vi "neuronFound.vi"(6 "Pipette broken threshold (MOhms)":dbl=-0.5, 8 "NH method":T1, 9 "Extra threshold (MOhms)":dbl=0.15, 10 "Detection Threshold (MOhms)":dbl=0.05, 11 "R array":dbl[](array[numeric])) -> (2 "pipette broken - abort!":bool, 3 "neuron found":bool)   [LabVIEW 2015]
uses:
  <vilib>/Analysis/NI_AALBase.lvlib
  <vilib>/Analysis/baseanly.llb/Mean (DBL).vi
  controls/NH_method.ctl
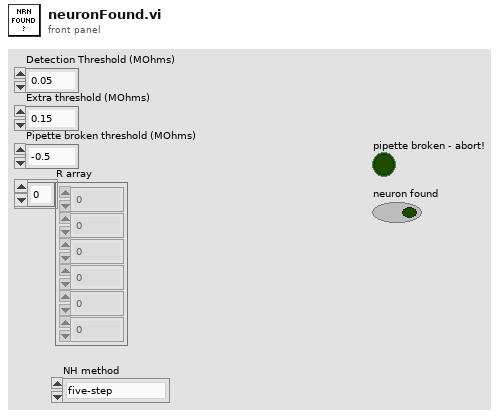
[diagram p1: front panel]
types:
  T1 = typedef "NH_method.ctl" = enum16{"five-step", "three-stepANDfixedCutOff", "three-step"}
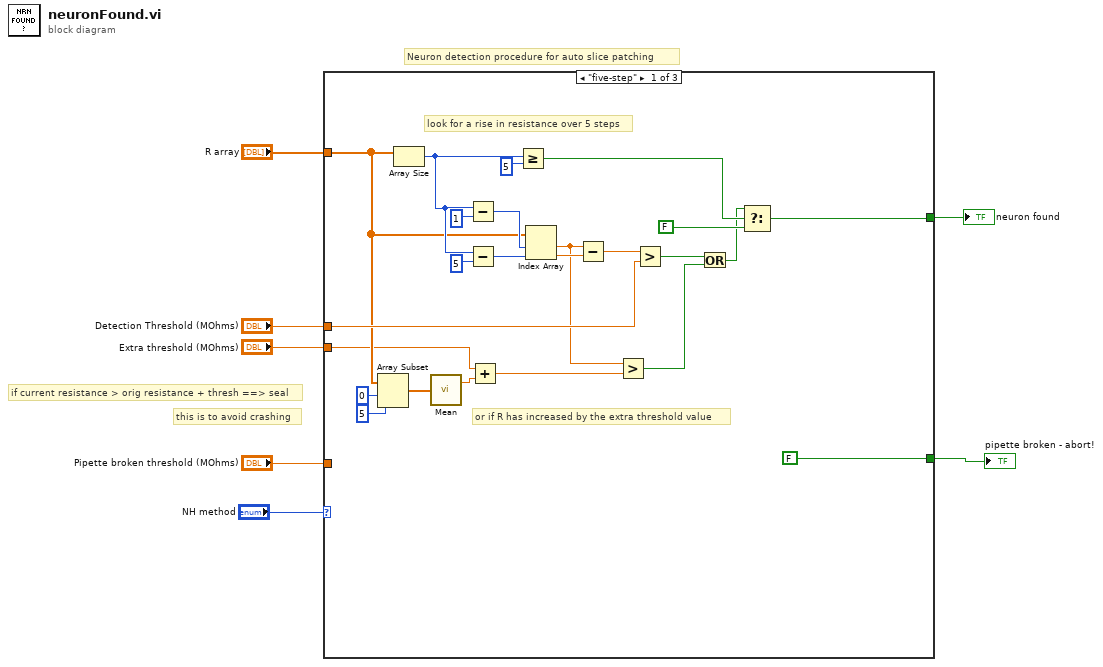
[diagram p0: block diagram]
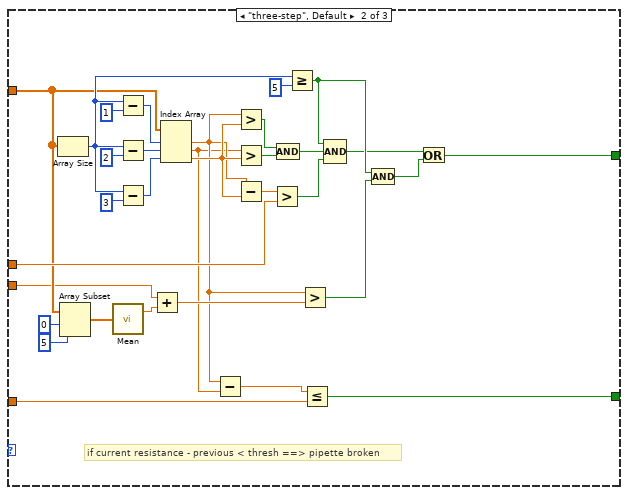
[diagram p2: hidden frame]
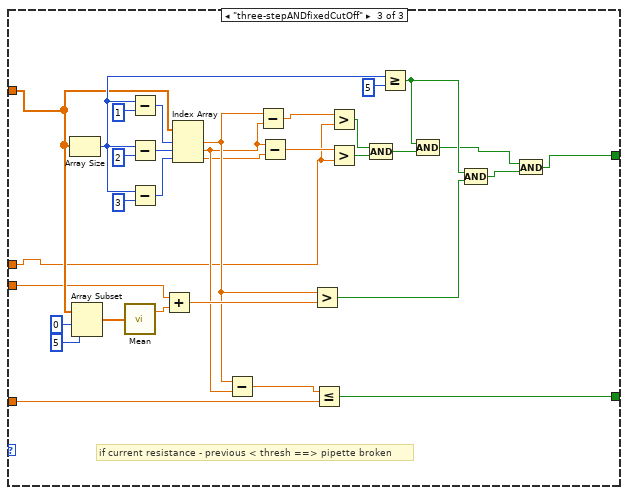
[diagram p3: hidden frame]
diagram:
  # "this is to avoid crashing"
  # "if current resistance > orig resistance + thresh ==> seal"
  # "Neuron detection procedure for auto slice patching"
  n1 = case shown="\"five-step\"" "NH method" {
    tunnel: [w20 w39 w64] -> w7
    tunnel: "R array" -> [w13 w48 w75]
    tunnel: "Detection Threshold (MOhms)" -> [w22 w63 w67]
    tunnel: "Extra threshold (MOhms)" -> [w8 w43 w74]
    tunnel: "Pipette broken threshold (MOhms)" -> [_ w33 w73]
    tunnel: [FALSE w32 w76] -> w1
    frame "five-step" {
      # "or if R has increased by the extra threshold value"
      # "look for a rise in resistance over 5 steps"
      n2 = Array Subset(array=w13, index=0, length=5) -> (w14:dbl[])
      n3 = Array Size(array=w13) -> (size(s)=w26:i32)
      n4 = call-poly <vilib>:"Mean.vi"("X"=w14) -> ("mean"=w16:dbl)  [unwired: 1 out]
      n5 = Subtract(x=w26, y=1) -> (x-y=w25:i32)
      n6 = Subtract(x=w26, y=5) -> (x-y=w21:i32)
      n7 = Add(x=w8, y=w16) -> (x+y=w15:dbl)
      n8 = Greater Or Equal?(x=w26, y=5) -> (x >= y?=w30:bool)
      n9 = Index Array(array=w13, index #1=w25, index #2=w21) -> (element #1=w11:dbl, element #2=w24:dbl)
      n10 = Subtract(x=w11, y=w24) -> (x-y=w23:dbl)
      n11 = Greater?(x=w11, y=w15) -> (0:w12:bool)
      n12 = Greater?(x=w23, y=w22) -> (0:w9:bool)
      n13 = Or(x=w9, y=w12) -> (x .or. y?=w10:bool)
      n14 = Select(t=w10, s=w30, f=FALSE) -> (s? t:f=w20:bool)
    }
    frame "three-step", Default {
      # "if current resistance - previous < thresh ==> pipette broken"
      n15 = Array Size(array=w48) -> (size(s)=w49:i32)
      n16 = Array Subset(array=w48, index=0, length=5) -> (w45:dbl[])
      n17 = call-poly <vilib>:"Mean.vi"("X"=w45) -> ("mean"=w44:dbl)  [unwired: 1 out]
      n18 = Subtract(x=w49, y=1) -> (x-y=w59:i32)
      n19 = Subtract(x=w49, y=2) -> (x-y=w58:i32)
      n20 = Subtract(x=w49, y=3) -> (x-y=w54:i32)
      n21 = Add(x=w43, y=w44) -> (x+y=w42:dbl)
      n22 = Index Array(array=w48, index #1=w59, index #2=w58, index #3=w54) -> (element #1=w36:dbl, element #2=w35:dbl, element #3=w50:dbl)
      n23 = Subtract(x=w36, y=w35) -> (x-y=w34:dbl)
      n24 = Greater?(x=w36, y=w50) -> (0:w53:bool)
      n25 = Greater?(x=w35, y=w50) -> (0:w52:bool)
      n26 = Subtract(x=w36, y=w50) -> (x-y=w56:dbl)
      n27 = Greater?(x=w56, y=w63) -> (0:w55:bool)
      n28 = Compound Arithmetic op=AND(w53, w52) -> (w51:bool)
      n29 = Greater Or Equal?(x=w49, y=5) -> (x >= y?=w41:bool)
      n30 = Greater?(x=w36, y=w42) -> (0:w37:bool)
      n31 = Less Or Equal?(x=w34, y=w33) -> (x <= y?=w32:bool)
      n32 = Compound Arithmetic op=AND(w41, w51, w55) -> (w40:bool)
      n33 = Compound Arithmetic op=AND(w41, w37) -> (w38:bool)
      n34 = Or(x=w40, y=w38) -> (x .or. y?=w39:bool)
    }
    frame "three-stepANDfixedCutOff" {
      # "if current resistance - previous < thresh ==> pipette broken"
      n35 = Array Size(array=w75) -> (size(s)=w85:i32)
      n36 = Array Subset(array=w75, index=0, length=5) -> (w82:dbl[])
      n37 = call-poly <vilib>:"Mean.vi"("X"=w82) -> ("mean"=w81:dbl)  [unwired: 1 out]
      n38 = Subtract(x=w85, y=1) -> (x-y=w92:i32)
      n39 = Subtract(x=w85, y=2) -> (x-y=w91:i32)
      n40 = Subtract(x=w85, y=3) -> (x-y=w89:i32)
      n41 = Add(x=w74, y=w81) -> (x+y=w80:dbl)
      n42 = Index Array(array=w75, index #1=w92, index #2=w91, index #3=w89) -> (element #1=w72:dbl, element #2=w71:dbl, element #3=w70:dbl)
      n43 = Subtract(x=w72, y=w71) -> (x-y=w77:dbl)
      n44 = Subtract(x=w72, y=w71) -> (x-y=w69:dbl)
      n45 = Subtract(x=w71, y=w70) -> (x-y=w68:dbl)
      n46 = Greater?(x=w72, y=w80) -> (0:w78:bool)
      n47 = Less Or Equal?(x=w77, y=w73) -> (x <= y?=w76:bool)
      n48 = Greater?(x=w69, y=w67) -> (0:w88:bool)
      n49 = Greater?(x=w68, y=w67) -> (0:w87:bool)
      n50 = Compound Arithmetic op=AND(w88, w87) -> (w86:bool)
      n51 = Greater Or Equal?(x=w85, y=5) -> (x >= y?=w79:bool)
      n52 = Compound Arithmetic op=AND(w79, w86) -> (w66:bool)
      n53 = Compound Arithmetic op=AND(w79, w78) -> (w65:bool)
      n54 = And(x=w66, y=w65) -> (x .and. y?=w64:bool)
    }
  }
  "neuron found" <- w7
  "pipette broken - abort!" <- w1
